vi "Removal of CP (SubVI).vi"(1 "ch_output in":cdb[](array[numeric]), 2 "cp_length":i16) -> (0 "ch_output out":cdb[](array[numeric]))   [LabVIEW 2015]
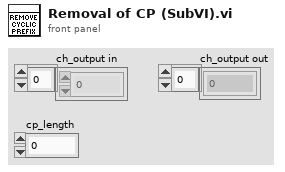
[diagram p1: front panel]
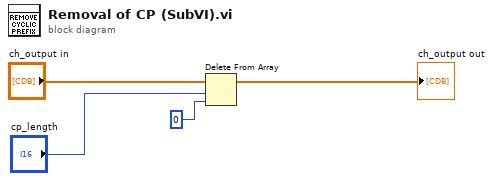
[diagram p0: block diagram]
diagram:
  n1 = Delete From Array(array="ch_output in", length="cp_length", index=0) -> (array with subset deleted=→"ch_output out":cdb[])  [unwired: 1 out]
